vi "ValidateIPorHostname.vi"(8 "error in (no error)":errorcluster, 11 "IP Address or Hostname":string) -> (0 "error out":errorcluster, 3 "Valid?":bool)   [LabVIEW 2021, in "myRIOMetaDataObj.lvclass"]
uses:
  myRIOMetaDataObj.lvclass
  <vilib>/Utility/error.llb/DialogType.ctl
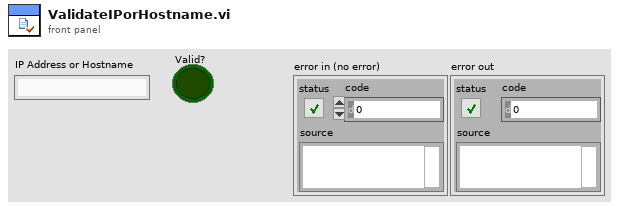
[diagram p1: front panel]
types:
  T1 = typedef "DialogType.ctl" = u16
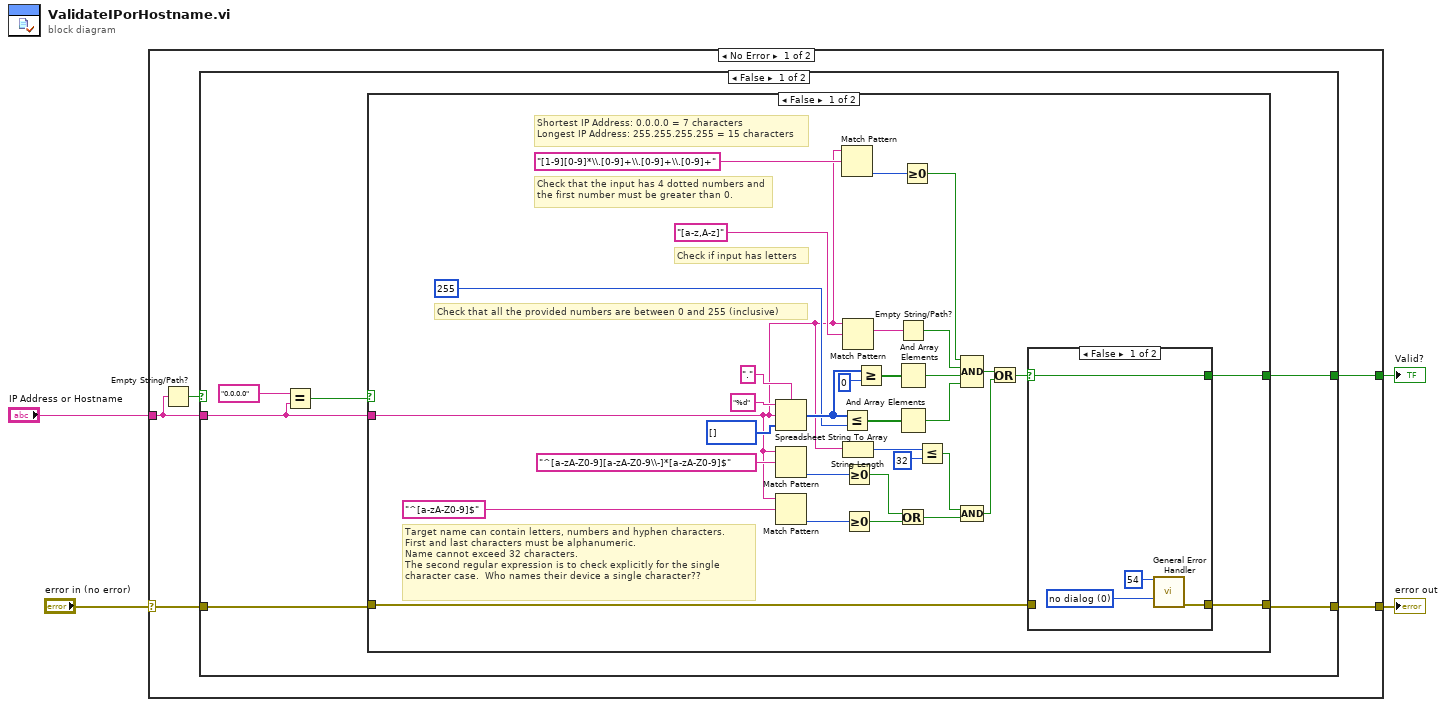
[diagram p0: block diagram]
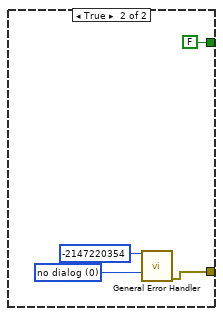
[diagram p3: hidden frame]
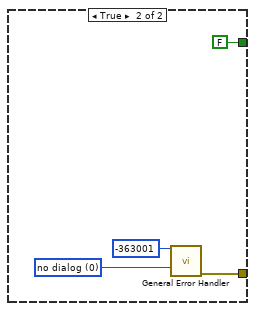
[diagram p4: hidden frame]
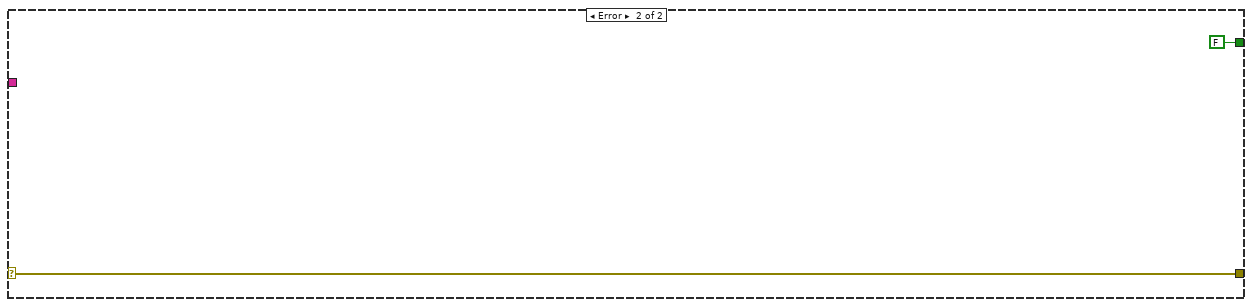
[diagram p5: hidden frame]
diagram:
  n1 = case shown="No Error" "error in (no error)" {
    selector: "error in (no error)" -> [w5 w64]
    tunnel: "IP Address or Hostname" -> [w8 _]
    tunnel: [w9 FALSE] -> w3
    tunnel: [w6 w64] -> w1
    frame No Error {
      n2 = Empty String/Path?(string/path=w8) -> (empty?=w7:bool)
      n3 = case shown="False" w7 {
        tunnel: w8 -> [w12 _]
        tunnel: [w15 FALSE] -> w9
        tunnel: [w13 w59] -> w6
        tunnel: w5 -> [w14 _]
        frame False {
          n4 = Equal?(x="0.0.0.0" ("false string"), y=w12) -> (x = y?=w10:bool)
          n5 = case shown="False" w10 {
            tunnel: w12 -> [w22 _]
            tunnel: [w21 FALSE] -> w15
            tunnel: w14 -> [w20 _]
            tunnel: [w19 w55] -> w13
            frame False {
              # "Target name can contain letters, numbers and hyphen characters. \nFirst and last characters must be alphanumeric.\nName cannot exceed 32 characters.\nThe second regular expression is to check explicitly for the single\ncharacter case.  Who names their device a single character??"
              # "Check that all the provided numbers are between 0 and 255 (inclusive)"
              # "Check if input has letters"
              # "Check that the input has 4 dotted numbers and the first number must be greater than 0."
              # "Shortest IP Address: 0.0.0.0 = 7 characters\nLongest IP Address: 255.255.255.255 = 15 characters"
              n6 = Spreadsheet String To Array(delimiter (Tab)=".", format string="%d", spreadsheet string=w22, array type (2D Dbl)=i32[] []) -> (array=w42:i32[])
              n7 = Match Pattern(string=w22, regular expression="^[a-zA-Z0-9][a-zA-Z0-9\\-]*[a-zA-Z0-9]$") -> (offset past match=w29:i32)  [unwired: 1 in, 3 out]
              n8 = Match Pattern(string=w22, regular expression="^[a-zA-Z0-9]$") -> (offset past match=w26:i32)  [unwired: 1 in, 3 out]
              n9 = Match Pattern(string=w22, regular expression="[1-9][0-9]*\\.[0-9]+\\.[0-9]+\\.[0-9]+") -> (offset past match=w37:i32)  [unwired: 1 in, 3 out]
              n10 = Less Or Equal?(x=w42, y=255) -> (x <= y?=w39:bool[])
              n11 = Match Pattern(string=w22, regular expression="[a-z,A-z]") -> (match substring=w38:string)  [unwired: 1 in, 3 out]
              n12 = String Length(string=w22) -> (length=w32:i32)
              n13 = Greater Or Equal To 0?(x=w29) -> (x >= 0?=w24:bool)
              n14 = Greater Or Equal To 0?(x=w26) -> (x >= 0?=w25:bool)
              n15 = Greater Or Equal?(x=w42, y=0) -> (x >= y?=w40:bool[])
              n16 = Empty String/Path?(string/path=w38) -> (empty?=w35:bool)
              n17 = And Array Elements(Boolean array=w40) -> (logical AND=w34:bool)
              n18 = And Array Elements(Boolean array=w39) -> (logical AND=w33:bool)
              n19 = Or(x=w24, y=w25) -> (x .or. y?=w23:bool)
              n20 = Greater Or Equal To 0?(x=w37) -> (x >= 0?=w36:bool)
              n21 = Less Or Equal?(x=w32, y=32) -> (x <= y?=w28:bool)
              n22 = Compound Arithmetic op=AND(w36, w35, w34, w33) -> (w17:bool)
              n23 = Compound Arithmetic op=AND(w28, w23) -> (w16:bool)
              n24 = Or(x=w17, y=w16) -> (x .or. y?=w18:bool)
              n25 = case shown="False" w18 {
                selector: w18 -> [w49 w54]
                tunnel: [w49 w54] -> w21
                tunnel: w20 -> [_ w53]
                tunnel: [w50 w53] -> w19
                frame False {
                  w51 = T1 0 items=["no dialog", "OK message", "continue or stop message", "OK message + warnings", "continue/stop + warnings"] ("type of dialog (OK msg:1)")
                  n26 = call <vilib>:"General Error Handler.vi"("[error code] (0)"=54, "type of dialog (OK msg:1)"=w51) -> ("error out"=w50:errorcluster)  [unwired: 9 in, 4 out]
                }
                frame True {
                }
              }
            }
            frame True {
              w57 = T1 0 items=["no dialog", "OK message", "continue or stop message", "OK message + warnings", "continue/stop + warnings"] ("type of dialog (OK msg:1)")
              n27 = call <vilib>:"General Error Handler.vi"("[error code] (0)"=-2147220354, "type of dialog (OK msg:1)"=w57) -> ("error out"=w55:errorcluster)  [unwired: 9 in, 4 out]
            }
          }
        }
        frame True {
          w60 = T1 0 items=["no dialog", "OK message", "continue or stop message", "OK message + warnings", "continue/stop + warnings"] ("type of dialog (OK msg:1)")
          n28 = call <vilib>:"General Error Handler.vi"("[error code] (0)"=-363001, "type of dialog (OK msg:1)"=w60) -> ("error out"=w59:errorcluster)  [unwired: 9 in, 4 out]
        }
      }
    }
    frame Error {
    }
  }
  "Valid?" <- w3
  "error out" <- w1
